vi "RGB_To_Colour_Box_Array.vi"(1 "Blue":dbl[][](array[numeric]), 2 "Green":dbl[][](array[numeric]), 3 "Red":dbl[][](array[numeric])) -> (0 "Colour Box":u32[][](array[colorbox]))   [LabVIEW 2016]
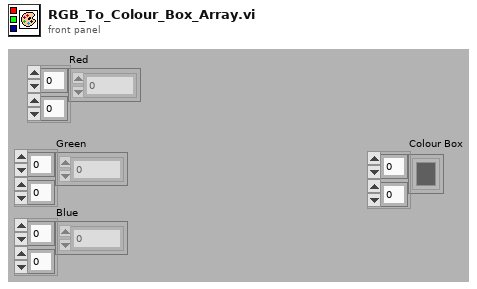
[diagram p1: front panel]
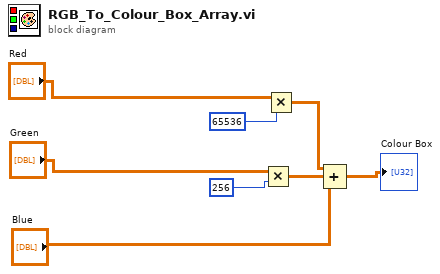
[diagram p0: block diagram]
diagram:
  n1 = Multiply(x="Green", y=256) -> (x*y=w5:dbl[][])
  n2 = Multiply(x="Red", y=65536) -> (x*y=w6:dbl[][])
  n3 = Compound Arithmetic op=ADD(w6, w5, "Blue") -> (→"Colour Box":dbl[][])
